vi "HIOKI PW3390 Configuration Simple Setting.vi"() -> ()   [LabVIEW 2009]
doc: "Sets the wiring mode and functions related to voltage and current."
uses:
  <instrlib>/PW3390/Common/_Initialize/HIOKI PW3390 Initialize LAN.vi
  <instrlib>/PW3390/Common/_Initialize/HIOKI PW3390 Initialize RS-232C.vi
panel:
  out "error out":errorcluster
  in  "Communication Interface":enum16{"LAN", "RS-232C"}(ring)
  in  "baud rate (38400bps)":u32=38400
  in  "COM Port":refnum<visa-resource-name>="COM1"
  in  "IP Address":string="192.168.1.1"
  in  "Wiring (0: 1P2W)":T1(ring)
  in  "Current":T2(array[cluster])=[{"Auto     "=FALSE, "Range       "=enum."500", "I rect"=FALSE}, {"Auto     "=FALSE, "Range       "=enum."500", "I rect"=FALSE}, {"Auto     "=FALSE, "Range       "=enum."500", "I rect"=FALSE}, {"Auto     "=FALSE, "Range       "=enum."500", "I rect"=FALSE}]
  in  "Voltage":T3(array[cluster])=[{"Auto     "=FALSE, "Range     "=enum."600", "U rect"=FALSE}, {"Auto     "=FALSE, "Range     "=enum."600", "U rect"=FALSE}, {"Auto     "=FALSE, "Range     "=enum."600", "U rect"=FALSE}, {"Auto     "=FALSE, "Range     "=enum."600", "U rect"=FALSE}]
  # "CH1"
  # "CH2"
  # "CH3"
  # "CH4"
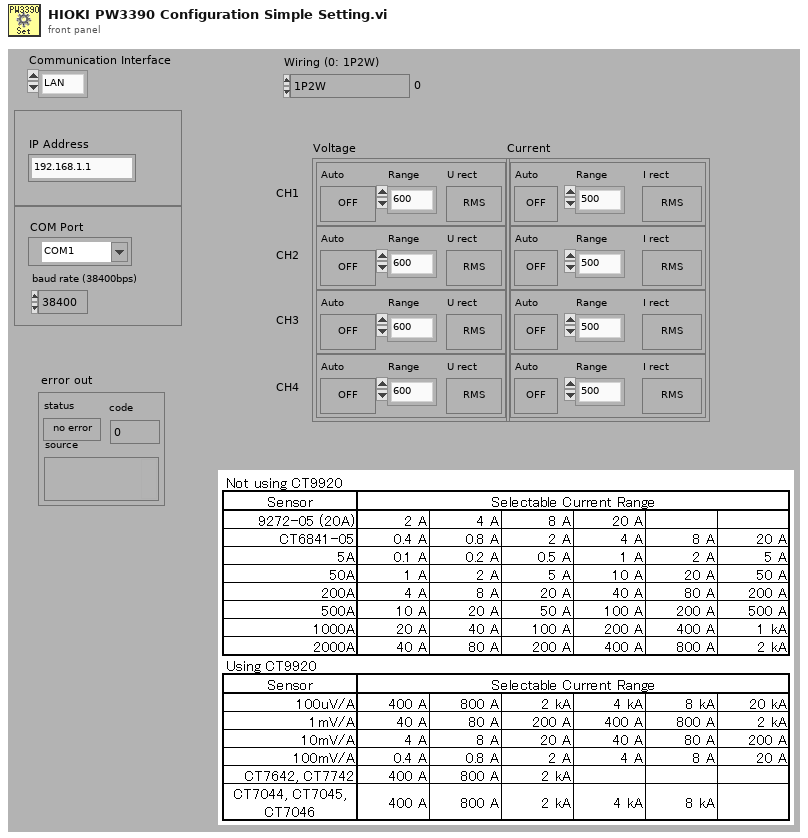
[diagram p1: front panel]
types:
  T1 = enum16{"1P2W", "1P3W, 1P2W", "3P3W2M, 1P2W", "1P3W, 1P3W", "3P3W2M, 1P3W", "3P3W2M, 3P3W2M", "3P3W3M, 1P2W", "3P4W, 1P2W"}
  T2 = cluster{"Auto     ":bool, "Range       ":enum16{"0.1", "0.2", "0.4", "0.5", "0.8", "1", "2", "4", "5", "8", "10", "20", "40", "50", "80", "100", "200", "400", "500", "800", "1000", "2000", "4000", "8000", "20000"}, "I rect":bool}[]
  T3 = cluster{"Auto     ":bool, "Range     ":enum16{"15", "30", "60", "150", "300", "600", "1500"}, "U rect":bool}[]
  T4 = enum16{"0.1", "0.2", "0.4", "0.5", "0.8", "1", "2", "4", "5", "8", "10", "20", "40", "50", "80", "100", "200", "400", "500", "800", "1000", "2000", "4000", "8000", "20000"}
  T5 = enum16{"15", "30", "60", "150", "300", "600", "1500"}
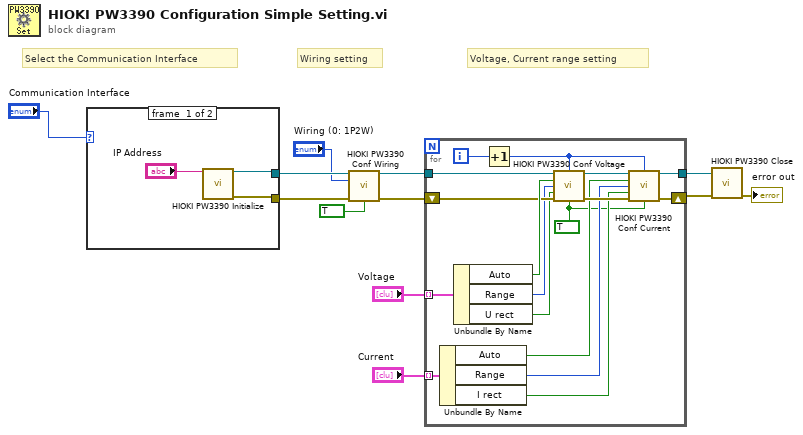
[diagram p0: block diagram]
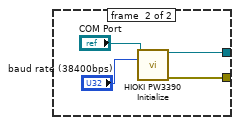
[diagram p2: hidden frame]
diagram:
  # "Select the Communication Interface"
  # "Voltage, Current range setting"
  # "Wiring setting"
  n1 = case shown="\"LAN\", デフォルト" "Communication Interface" {
    tunnel: [w14 w19] -> w10
    tunnel: [w13 w18] -> w9
    frame #0 {
      n2 = call-poly <instrlib>:"HIOKI PW3390 Initialize.vi"("IP Address"="IP Address") -> ("VISA Resource out"=w14:refnum<visa-resource-name>, "error out"=w13:errorcluster)  [unwired: 12 in, 1 out]
    }
    frame #1 {
      n3 = call-poly <instrlib>:"HIOKI PW3390 Initialize.vi"("COM Port"="COM Port", "baud rate (38400bps)"="baud rate (38400bps)") -> ("VISA Resource out"=w19:refnum<visa-resource-name>, "error out"=w18:errorcluster)  [unwired: 11 in, 1 out]
    }
  }
  n4 = call <instrlib>:"HIOKI PW3390 Conf Wiring.vi"("VISA Resource"=w10, "Wiring (0: 1P2W)"="Wiring (0: 1P2W)", "error in (no error)"=w9, "Error Out (F: Off)"=TRUE) -> ("VISA Resource out"=w7:refnum<visa-resource-name>, "error out"=w6:errorcluster)  [unwired: 9 in, 1 out]
  n5 = for {
    tunnel: "Voltage" -> [w36] mode=indexing
    tunnel: "Current" -> [w35] mode=indexing
    tunnel: w7 -> [w32]
    tunnel: [w23] -> w4
    shift-right: [w22] -> w3
    shift-left: w6 -> [w29]
    i -> [w21]
    w20 = TRUE ("Error Out (F: Off)")
    n6 = Unbundle By Name(w35) -> ("Auto"=w26:bool, "Range"=w25:T4, "I rect"=w24:bool)
    n7 = Unbundle By Name(w36) -> ("Auto"=w33:bool, "Range"=w28:T5, "U rect"=w27:bool)
    n8 = Increment(x=w21) -> (x+1=w34:i32)
    n9 = call <instrlib>:"HIOKI PW3390 Conf Voltage.vi"("VISA Resource"=w32, "CH (1)"=w34, "Auto (F: OFF)"=w33, "Range (5: 600V)"=w28, "U rect (F: RMS)"=w27, "error in (no error)"=w29, "Error Out (F: Off)"=w20) -> ("VISA Resource out"=w31:refnum<visa-resource-name>, "error out"=w30:errorcluster)  [unwired: 4 in, 3 out]
    n10 = call <instrlib>:"HIOKI PW3390 Conf Current.vi"("VISA Resource"=w31, "CH (1)"=w34, "Auto (F: OFF)"=w26, "Range (18: 500A)"=w25, "I rect (F: RMS)"=w24, "error in (no error)"=w30, "Error Out (F: Off)"=w20) -> ("VISA Resource out"=w23:refnum<visa-resource-name>, "error out"=w22:errorcluster)  [unwired: 4 in, 3 out]
  }
  n11 = call <instrlib>:"HIOKI PW3390 Close.vi"("VISA Resource"=w4, "error in (no error)"=w3) -> ("error out"=→"error out":errorcluster)  [unwired: 13 in]
